vi "fuenteVoltajenueva.vi"(8 "entrada":dbl min=-210.0 max=210.0, 9 "Source Mode  (0: Voltage)":u16(ring) items=["Voltage", "Current"], 11 "VISA resource name":refnum<visa-resource-name>) -> (1 "CORRIENTE":dbl, 2 "VOLTAJE":dbl)   [LabVIEW 2016]
uses:
  <instrlib>/Keithley 2450/Keithley 2450.lvlib
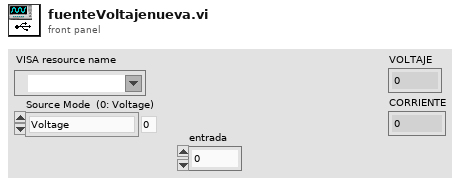
[diagram p1: front panel]
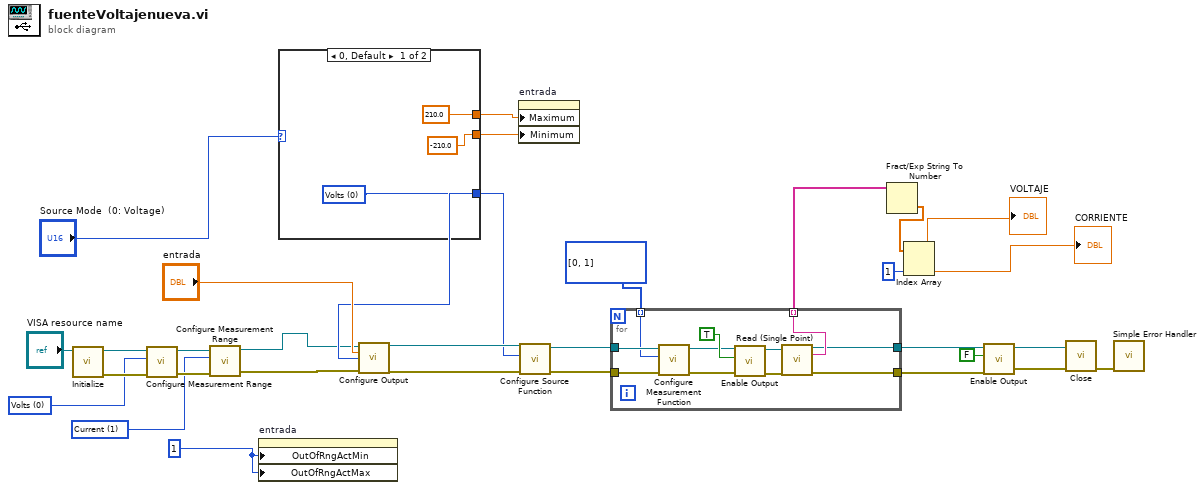
[diagram p0: block diagram]
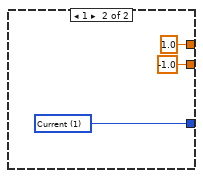
[diagram p2: hidden frame]
diagram:
  w1 = u8 1 ("Response to Value Outside Limits:Minimum")
  w18 = u16[] [0, 1] items=["Volts", "Current", "Auto Resistance", "Manual Resistance", "Digitize Voltage", "Digitize Current"]
  w25 = u16 1 items=["Volts", "Current", "Resistance"] ("Function (0: Volts)")
  w28 = u16 0 items=["Volts", "Current", "Resistance"] ("Function (0: Volts)")
  n1 = call <instrlib>:"Initialize.vi"("VISA resource name"="VISA resource name") -> ("error out"=w30:errorcluster, "VISA resource name out"=w31:refnum<visa-resource-name>)  [unwired: 9 in]
  n2 = call <instrlib>:"Configure Measurement Range.vi"("error in (no error)"=w30, "Function (0: Volts)"=w28, "VISA resource name"=w31) -> ("error out"=w26:errorcluster, "VISA resource name out"=w27:refnum<visa-resource-name>)  [unwired: 7 in]
  n3 = call <instrlib>:"Configure Measurement Range.vi"("error in (no error)"=w26, "Function (0: Volts)"=w25, "VISA resource name"=w27) -> ("error out"=w5:errorcluster, "VISA resource name out"=w6:refnum<visa-resource-name>)  [unwired: 7 in]
  n4 = property on="entrada" class="DigNum (strict)"("OutOfRngActMin"=w1, "OutOfRngActMax"=w1) -> ()  [unwired: 2 in, 2 out]
  n5 = case shown="0, Default" "Source Mode  (0: Voltage)" {
    tunnel: [w34 w37] -> w21
    tunnel: [210.0 1.0] -> w3
    tunnel: [-210.0 -1.0] -> w2
    frame 0, Default {
      w34 = u16 0 items=["Volts", "Current"] ("Function (0: Volts)")
    }
    frame 1 {
      w37 = u16 1 items=["Volts", "Current"] ("Function (0: Volts)")
    }
  }
  n6 = call <instrlib>:"Configure Output.vi"("VISA resource name"=w6, "Source Level (0)"="entrada", "Source Mode  (0: Voltage)"=w21, "error in (no error)"=w5) -> ("VISA resource name out"=w23:refnum<visa-resource-name>, "error out"=w22:errorcluster)  [unwired: 10 in]
  n7 = property on="entrada" class="DigNum (strict)"("Maximum"=w3, "Minimum"=w2) -> ()  [unwired: 2 in, 2 out]
  n8 = call <instrlib>:"Configure Source Function.vi"("error in (no error)"=w22, "Function (0: Volts)"=w21, "VISA resource name"=w23) -> ("error out"=w19:errorcluster, "VISA resource name out"=w20:refnum<visa-resource-name>)  [unwired: 7 in]
  n9 = for {
    tunnel: w20 -> [w48]
    tunnel: w19 -> [w47]
    tunnel: [w46] -> w17 mode=indexing
    tunnel: [w45] -> w12
    tunnel: [w44] -> w11
    tunnel: w18 -> [w43] mode=indexing
    n10 = call <instrlib>:"Configure Measurement Function.vi"("error in (no error)"=w47, "Function (0: Volts)"=w43, "VISA resource name"=w48) -> ("error out"=w40:errorcluster, "VISA resource name out"=w41:refnum<visa-resource-name>)  [unwired: 7 in]
    n11 = call <instrlib>:"Enable Output.vi"("error in (no error)"=w40, "Enable Output (T: Enable)"=TRUE, "VISA resource name"=w41) -> ("error out"=w39:errorcluster, "VISA resource name out"=w38:refnum<visa-resource-name>)  [unwired: 7 in]
    n12 = call <instrlib>:"Read (Single Point).vi"("VISA resource name"=w38, "error in (no error)"=w39) -> ("VISA resource name out"=w45:refnum<visa-resource-name>, "Data out"=w46:string, "error out"=w44:errorcluster)  [unwired: 11 in]
  }
  n13 = Fract/Exp String To Number(string=w17) -> (number=w16:dbl[])  [unwired: 3 in, 1 out]
  n14 = Index Array(array=w16, index #2=1 ("index")) -> (element #1=→"VOLTAJE":dbl, element #2=→"CORRIENTE":dbl)  [unwired: 1 in]
  n15 = call <instrlib>:"Enable Output.vi"("error in (no error)"=w11, "Enable Output (T: Enable)"=FALSE, "VISA resource name"=w12) -> ("error out"=w8:errorcluster, "VISA resource name out"=w9:refnum<visa-resource-name>)  [unwired: 7 in]
  n16 = call <instrlib>:"Close.vi"("error in (no error)"=w8, "VISA resource name"=w9) -> ("error out"=w10:errorcluster)  [unwired: 9 in]
  n17 = call <vilib>:"Simple Error Handler.vi"("error in (no error)"=w10) -> ()  [unwired: 4 in, 5 out]
